vi "timestampManifest.set.vi"(8 "error in (no error)":errorcluster, 10 "nominal types.lvlib:timestampManifest.lvlib:timestampManifest.lvclass":refnum<class "timestampManifest.lvclass">, 11 "video in":refnum<class "video.lvclass">) -> (0 "error out":errorcluster, 3 "video out":refnum<class "video.lvclass">)   [LabVIEW 2020, in "datasources.lvlib" / "video.lvclass"]
uses:
  video.lvclass
  nominal types/timestampManifest/timestampManifest/timestampManifest.lvclass
  video.lvclass/video.ctl
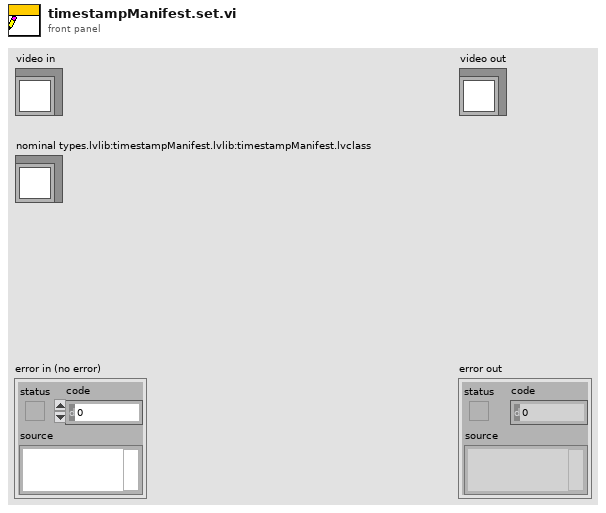
[diagram p1: front panel]
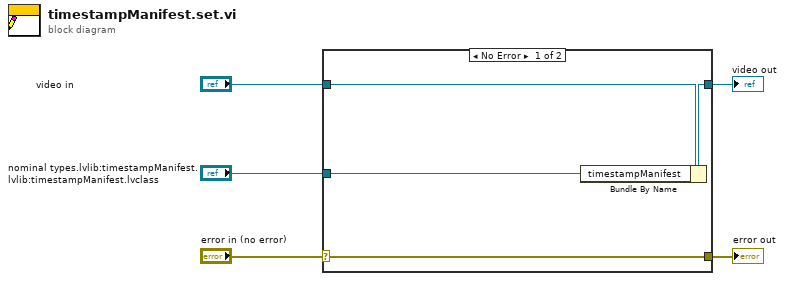
[diagram p0: block diagram]
diagram:
  n1 = case shown="No Error" "error in (no error)" {
    selector: "error in (no error)" -> [w9 w10]
    tunnel: [w9 w10] -> w4
    tunnel: [w7 w11] -> w2
    tunnel: "video in" -> [w8 w11]
    tunnel: "nominal types.lvlib:timestampManifest.lvlib:timestampManifest.lvclass" -> [w6 _]
    frame No Error {
      n2 = Bundle By Name(cluster=w8, "timestampManifest"=w6) -> (w7:refnum<class "video.lvclass">)
    }
    frame Error {
    }
  }
  "error out" <- w4
  "video out" <- w2
